vi "ManualMove.vi"() -> ()   [LabVIEW 2017]
panel:
  in  "Motor 2 Encoder Target":i32(slide) scale=-100.0..100.0
  in  "Motor 1 Encoder Target":i32(slide) scale=-100.0..100.0
  out "Battery Voltage Output":u16
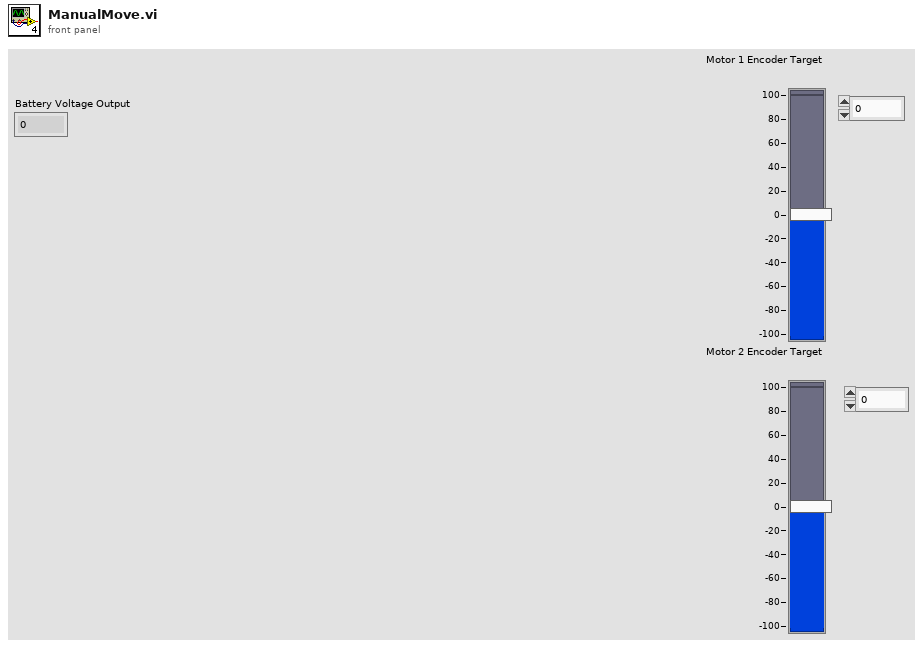
[diagram p1: front panel]
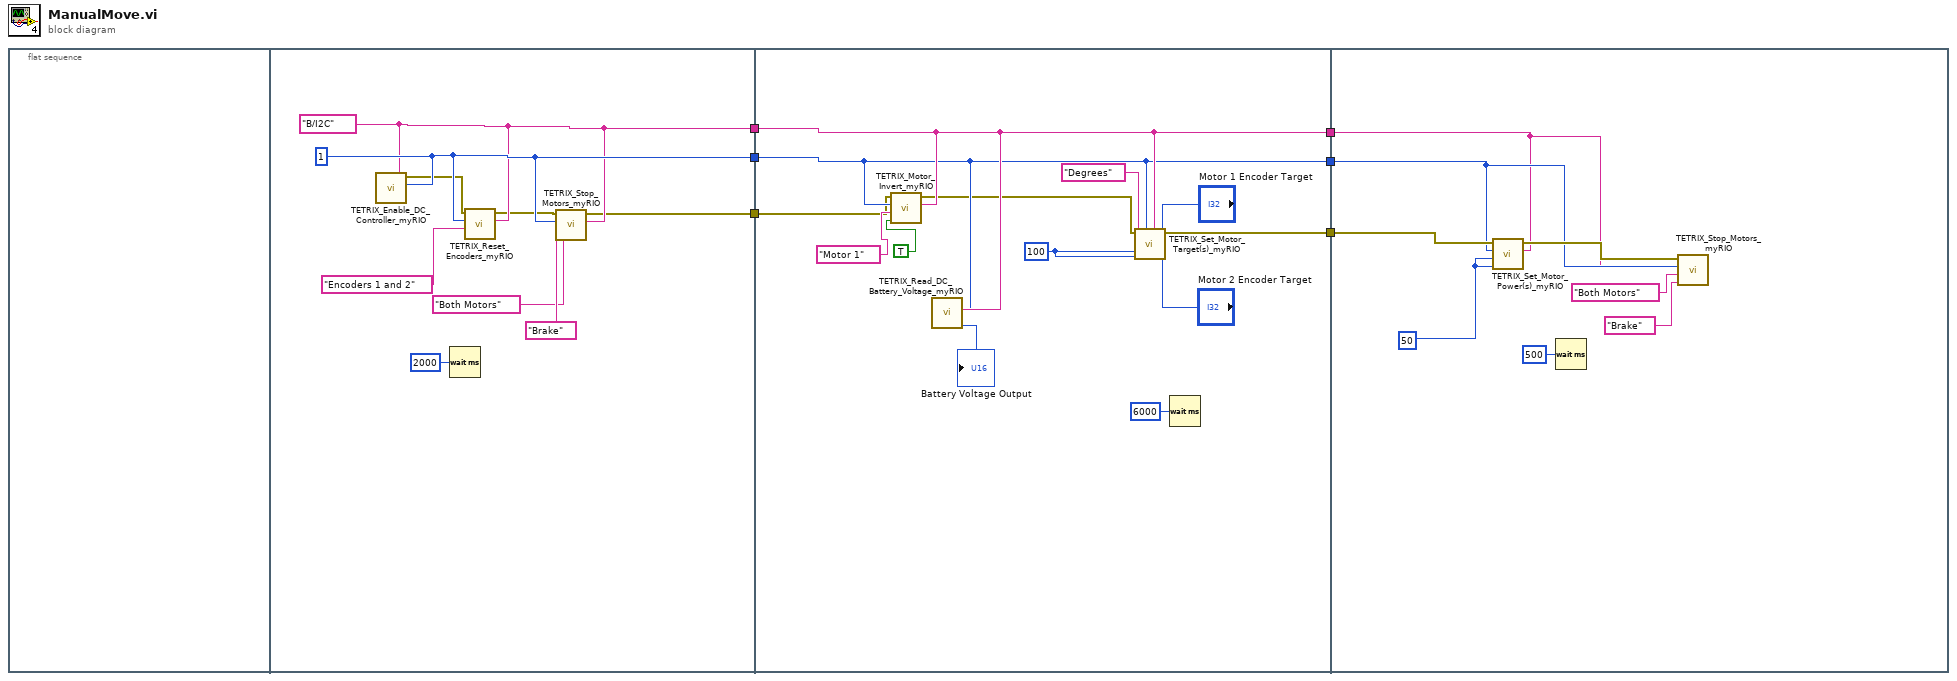
[diagram p0: block diagram]
diagram:
  n1 = flat-sequence {
    tunnel: [w11] -> w6
    tunnel: [w10] -> w5
    tunnel: [w7] -> w2
    tunnel: w6 -> [w19]
    tunnel: w5 -> [w20]
    tunnel: [w20] -> w4
    tunnel: [w19] -> w3
    tunnel: w2 -> [w18]
    tunnel: [w16] -> w1
    tunnel: w4 -> [w30]
    tunnel: w3 -> [w31]
    tunnel: w1 -> [w33]
    frame #0 {
    }
    frame #1 {
      w10 = tag "B/I2C" ("myRIO MXP Port A/B")
      w11 = u8 1 ("Controller ID#  (I2C Address)")
      n2 = call <vilib>:"TETRIX_Enable_DC_Controller_myRIO.vi"("myRIO MXP Port A/B"=w10, "Controller ID#  (I2C Address)"=w11) -> ("Error/Flow Out"=w9:errorcluster)  [unwired: 5 in]
      n3 = Wait (ms)(milliseconds to wait=u32 2000) -> ()  [unwired: 1 out]
      n4 = call <vilib>:"TETRIX_Reset_Encoders_myRIO.vi"("myRIO MXP Port A/B"=w10, "Select Encoder"="Encoders 1 and 2", "Controller ID#  (I2C Address)"=w11, "Error/Flow In"=w9) -> ("Error/Flow Out"=w8:errorcluster)  [unwired: 3 in]
      n5 = call <vilib>:"TETRIX_Stop_Motors_myRIO.vi"("myRIO MXP Port A/B"=w10, "Stop Mode"="Brake", "Select Channel"="Both Motors", "Controller ID#  (I2C Address)"=w11, "Error/Flow In"=w8) -> ("Error/Flow Out"=w7:errorcluster)  [unwired: 2 in]
    }
    frame #2 {
      w26 = i16 100 ("Motor 1 Contant Speed (Degrees per Second)")
      n6 = call <vilib>:"TETRIX_Motor_Invert_myRIO.vi"("myRIO MXP Port A/B"=w20, "Invert State"=TRUE, "Select Channel"="Motor 1", "Controller ID#  (I2C Address)"=w19, "Error/Flow In"=w18) -> ("Error/Flow Out"=w17:errorcluster)  [unwired: 2 in]
      n7 = call <vilib>:"TETRIX_Read_DC_Battery_Voltage_myRIO.vi"("myRIO MXP Port A/B"=w20, "Controller ID#  (I2C Address)"=w19) -> ("Battery Voltage Output"=→"Battery Voltage Output":u16)  [unwired: 4 in, 1 out]
      n8 = call <vilib>:"TETRIX_Set_Motor_Target(s)_myRIO.vi"("Motor 2 Encoder Target"="Motor 2 Encoder Target", "Motor 1 Encoder Target"="Motor 1 Encoder Target", "myRIO MXP Port A/B"=w20, "Controller ID#  (I2C Address)"=w19, "Motor 2 Constant Speed (Degrees per Second)"=w26, "Motor 1 Contant Speed (Degrees per Second)"=w26, "Encoder Units"="Degrees", "Error/Flow In"=w17) -> ("Error/Flow Out"=w16:errorcluster)  [unwired: 1 in]
      n9 = Wait (ms)(milliseconds to wait=u32 6000) -> ()  [unwired: 1 out]
    }
    frame #3 {
      w29 = i8 50 ("Motor 1 Power (-100 to 100)  0 = Coast Stop  125 = Brake Stop")
      n10 = call <vilib>:"TETRIX_Set_Motor_Power(s)_myRIO.vi"("myRIO MXP Port A/B"=w30, "Motor 2 Power (-100 to 100)  0 = Coast Stop  125 = Brake Stop"=w29, "Motor 1 Power (-100 to 100)  0 = Coast Stop  125 = Brake Stop"=w29, "Controller ID#  (I2C Address)"=w31, "Error/Flow In"=w33) -> ("Error/Flow Out"=w32:errorcluster)  [unwired: 2 in]
      n11 = Wait (ms)(milliseconds to wait=u32 500) -> ()  [unwired: 1 out]
      n12 = call <vilib>:"TETRIX_Stop_Motors_myRIO.vi"("myRIO MXP Port A/B"=w30, "Stop Mode"="Brake", "Select Channel"="Both Motors", "Controller ID#  (I2C Address)"=w31, "Error/Flow In"=w32) -> ()  [unwired: 2 in, 1 out]
    }
  }
